vi "dsdll_open.vi"(7 "format":T1={"sample rate [Hz]"=48000, "out channels"=2, "inp channels"=32, "format"=enum."PCM 16 bit"}, 8 "error in":errorcluster, 9 "capture device id":i32=-1, 10 "output device id":i32=-1, 11 "dsdll instance in":T3={"dsdll path"=path "E:/LVprog/DirectSoundDLL/dsdll.dll", "dsdll handle"=[], "output devices"=[], "capture devices"=[]}) -> (0 "error out":errorcluster, 3 "dsdll instance out":T3)   [LabVIEW 2018, in "dsdll.lvlib"]
doc: "Call this to open output and capture DirectSound devices.\n\nThe devices are selected by the index of the item in the previously enumerated device lists (dsdll_enumerate.vi). If the device id is not connected the output/capture device will not be opened. The library will work even if only output or input is opened.\n\nFormat cluster specifies format of the output and capture stream. The sampling rate is common for capture and output device. The channel count must be always valid, i.e. 1 or 2 even if the capture/output device is not used!"
uses:
  dsdll.lvlib
  dsdll_instance.ctl
  dsdll_device_record.ctl
  dsdll_format.ctl
  dsdll_sample_format.ctl
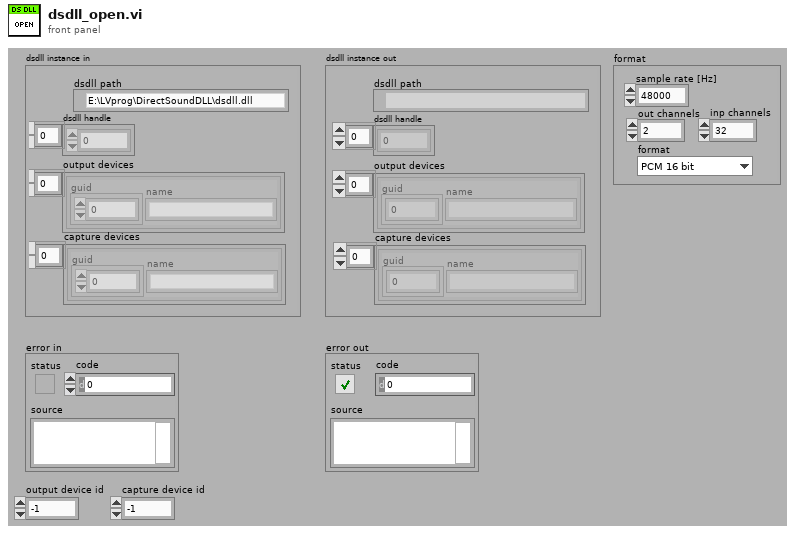
[diagram p1: front panel]
types:
  T1 = typedef "dsdll.lvlib/dsdll_format.ctl" = cluster{"sample rate [Hz]":u32, "out channels":u16, "inp channels":u16, "format":T2}
  T2 = typedef "dsdll.lvlib/dsdll_sample_format.ctl" = enum16{"IEEE float 32", "PCM 16 bit"}
  T3 = typedef "dsdll.lvlib/dsdll_instance.ctl" = cluster{"dsdll path":path, "dsdll handle":u8[], "output devices":T4[], "capture devices":T4[]}
  T4 = typedef "dsdll.lvlib/dsdll_device_record.ctl" = cluster{"guid":u8[], "name":string}
  T5 = enum16{"big-endian, network order", "native, host order", "little-endian"}
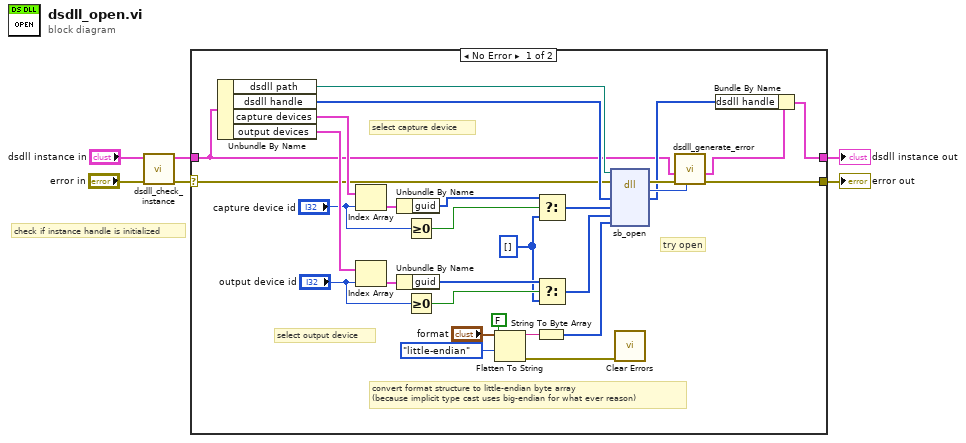
[diagram p0: block diagram]
diagram:
  # "check if instance handle is initialized"
  n1 = call "dsdll_check_instance.vi"("error in"="error in", "dsdll instance in"="dsdll instance in") -> ("error out"=w2:errorcluster, "dsdll instance out"=w1:T3)  [unwired: 7 in, 1 out]
  n2 = case shown="No Error" w2 {
    selector: w2 -> [w17 w36]
    tunnel: w1 -> [w18 w37]
    tunnel: [w27 w36] -> w3
    tunnel: [w25 w37] -> w4
    frame No Error {
      w20 = u8[] []
      # "convert format structure to little-endian byte array\n(because implicit type cast uses big-endian for what ever reason)"
      # "select output device"
      # "select capture device"
      # "try open"
      n3 = Unbundle By Name(w18) -> ("dsdll path"=w33:path, "dsdll handle"=w32:u8[], "capture devices"=w31:T4[], "output devices"=w28:T4[])
      n4 = Index Array(array=w31, index="capture device id") -> (element=w30:T4)
      n5 = Index Array(array=w28, index="output device id") -> (element=w29:T4)
      n6 = Unbundle By Name(w30) -> ("guid"=w23:u8[])
      n7 = Unbundle By Name(w29) -> ("guid"=w22:u8[])
      n8 = Greater Or Equal To 0?(x="capture device id") -> (x >= 0?=w24:bool)
      n9 = Greater Or Equal To 0?(x="output device id") -> (x >= 0?=w21:bool)
      n10 = Flatten To String(anything="format", prepend array or string size? (T)=FALSE, byte order (0:big-endian, network order)=T5."little-endian") -> (data string=w10:string, error out=w8:errorcluster)  [unwired: 1 in, 1 out]
      n11 = String To Byte Array(string=w10) -> (unsigned byte array=w9:u8[])
      n12 = Select(t=w23, s=w24, f=w20) -> (s? t:f=w16:u8[])
      n13 = Select(t=w22, s=w21, f=w20) -> (s? t:f=w15:u8[])
      n14 = dll-call lib="dsdll.dll" fn="sb_open" ("sb_get_handle_size()")(path in=w33, error in=w17, "handle"=w32, "input_guid"=w16, "output_guid"=w15, "format"=w9) -> (error out=w35:errorcluster, "error"=w34:i32, "handle"=w19:u8[])  [unwired: 4 in, 1 out]
      n15 = call <vilib>:"Clear Errors.vi"("error in (no error)"=w8) -> ()  [unwired: 5 in, 2 out]
      n16 = call "dsdll_generate_error.vi"("error code"=w34, "error in"=w35, "dsdll instance in"=w18) -> ("error out"=w27:errorcluster, "dsdll instance out"=w26:T3)  [unwired: 6 in, 1 out]
      n17 = Bundle By Name(cluster=w26, "dsdll handle"=w19) -> (w25:T3)
    }
    frame Error {
    }
  }
  "error out" <- w3
  "dsdll instance out" <- w4
